vi "Setup Grid Waypoint Params.vi"(9 "Grid Setup Complete?":bool, 10 "Virtual Waypoint":T3, 11 "Waypoints":T1[](array[typedef])) -> (2 "Grid Setup Complete? Out":bool, 3 "Waypoints Out":T1[](array[typedef]))   [LabVIEW 2014]
uses:
  Missions/Controls/Virtual Waypoint.ctl
  Missions/Controls/Waypoint Type.ctl
  Controls/Mission Planning Controls/MAVLINK Mission Item.ctl
  Controls/MAVLINK Mav Frame.ctl
  Commands/Mission Planning/MISSION_ITEM SubVI/MISSION_ITEM Set Camera Trigger Distance.vi
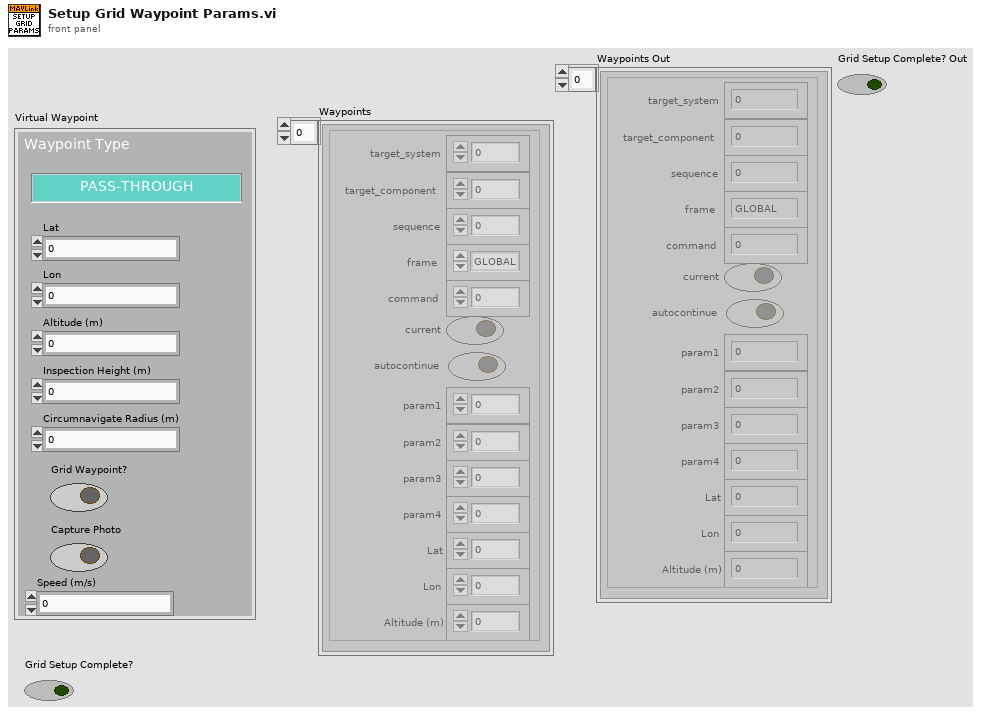
[diagram p1: front panel]
types:
  T1 = typedef "MAVLINK Mission Item.ctl" = cluster{"target_system":u8, "target_component":u8, "sequence":u16, "frame":T2, "command":u16, "current":bool, "autocontinue":bool, "param1":sgl, "param2":sgl, "param3":sgl, "param4":sgl, "Lat":sgl, "Lon":sgl, "Altitude (m)":sgl}
  T2 = typedef "MAVLINK Mav Frame.ctl" = enum8{"GLOBAL", "LOCAL NED", "MISSION", "GLOBAL RELATIVE ALT", "LOCAL ENU", "GLOBAL INT", "GLOBAL RELATIVE ALT INT", "LOCAL OFFSET NED", "BODY NED", "BODY OFFSET NED", "GLOBAL TERRAIN ALT", "GLOBAL TERRAIN ALT INT"}
  T3 = typedef "Virtual Waypoint.ctl" = cluster{"Waypoint Type":T4, "Lat":sgl, "Lon":sgl, "Altitude (m)":sgl, "Inspection Height (m)":sgl, "Circumnavigate Radius (m)":sgl, "Grid Waypoint?":bool, "Capture Photo":bool, "Speed (m/s)":sgl}
  T4 = typedef "Waypoint Type.ctl" = enum16{"PASS-THROUGH", "INSPECT", "CIRCUMNAVIGATE"}
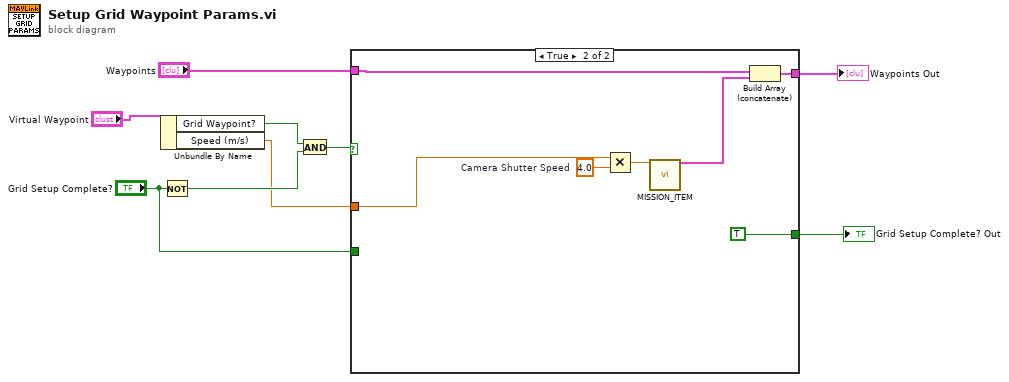
[diagram p0: block diagram]
diagram:
  n1 = Unbundle By Name("Virtual Waypoint") -> ("Grid Waypoint?"=w8:bool, "Speed (m/s)"=w4:sgl)
  n2 = Not(x="Grid Setup Complete?") -> (.not. x?=w7:bool)
  n3 = And(x=w8, y=w7) -> (x .and. y?=w6:bool)
  n4 = case shown="True" w6 {
    tunnel: "Waypoints" -> [w10 w15]
    tunnel: w4 -> [_ w14]
    tunnel: [w10 w13] -> w3
    tunnel: [w11 TRUE ("Grid Setup Complete? Out")] -> w2
    tunnel: "Grid Setup Complete?" -> [w11 _]
    frame False {
    }
    frame True {
      w17 = sgl 4.0  # Camera Shutter Speed
      n5 = Multiply(x=w14, y=w17) -> (x*y=w16:sgl)
      n6 = call-poly "MISSION_ITEM.vi"("Distance (m)"=w16) -> ("Mission Item"=w18:T1)  [unwired: 14 in]
      n7 = Build Array (concatenate)(w15, w18) -> (w13:T1[])
    }
  }
  "Waypoints Out" <- w3
  "Grid Setup Complete? Out" <- w2
